vi "CalculoSenoide.vi"(10 "InfoGeraOnda":T1, 11 "InfoOndaIn":cluster{"PontosOnda":dbl[], "IndexTemp":i32}) -> (3 "InfoOndaOut":cluster{"PontosOnda":dbl[], "IndexTemp":i32})   [LabVIEW 2019]
panel:
  # "Max: 60 pontos por segundo"
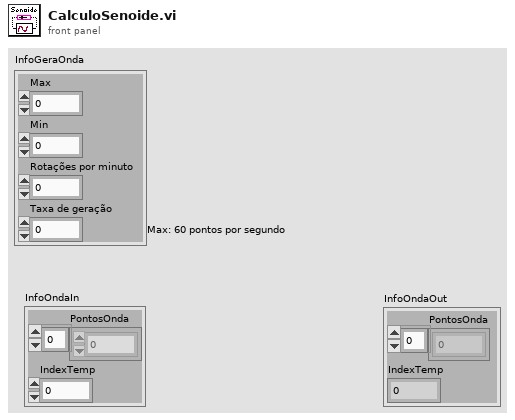
[diagram p1: front panel]
types:
  T1 = cluster{"Max":dbl, "Min":dbl, "Rotações por minuto":dbl, "Taxa de geração":dbl}
  T2 = cluster{"RotaçãoPorSeg":dbl, "Fase":dbl, "AmplitudeOnda":dbl, "Offset":dbl}
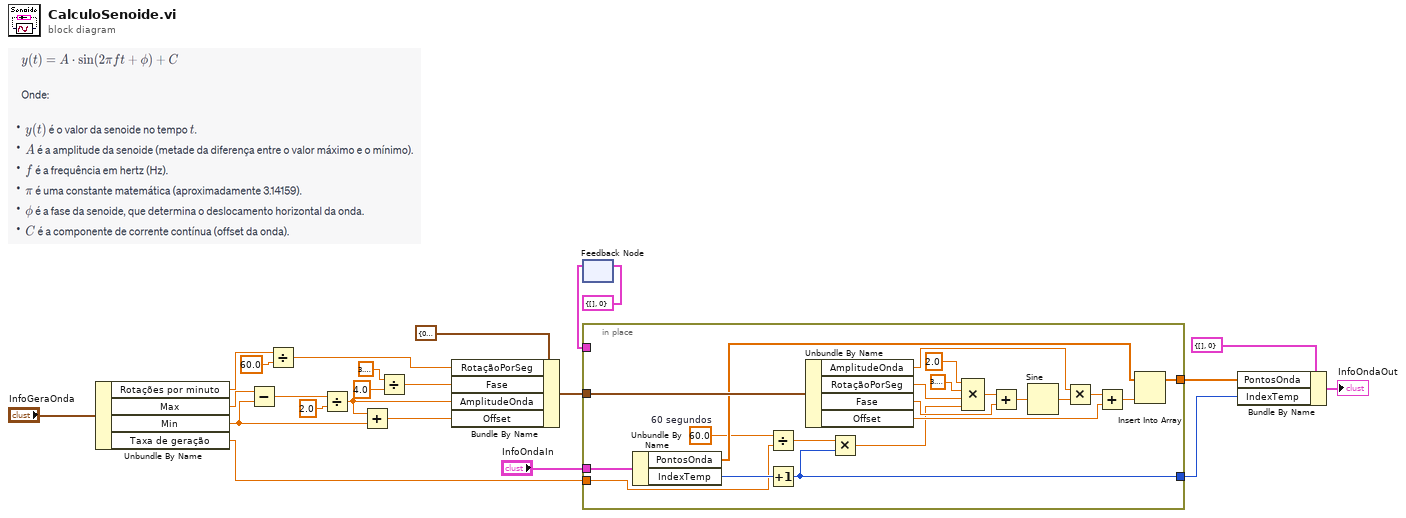
[diagram p0: block diagram]
diagram:
  n1 = Unbundle By Name("InfoGeraOnda") -> ("Rotações por minuto"=w4:dbl, "Max"=w3:dbl, "Min"=w2:dbl, "Taxa de geração"=w1:dbl)
  n2 = Subtract(x=w3, y=w2) -> (x-y=w19:dbl)
  n3 = Divide(x=w4, y=60.0) -> (x/y=w17:dbl)
  n4 = Divide(x=w19, y=2.0) -> (x/y=w15:dbl)
  n5 = Add(x=w15, y=w2) -> (x+y=w14:dbl)
  n6 = Divide(x=3.141592653589793, y=4.0) -> (x/y=w16:dbl)
  n7 = Bundle By Name(cluster=T2 {"RotaçãoPorSeg"=0.0, "Fase"=0.0, "AmplitudeOnda"=0.0, "Offset"=0.0}, "RotaçãoPorSeg"=w17, "Fase"=w16, "AmplitudeOnda"=w15, "Offset"=w14) -> (w13:T2)
  n8 = feedback #1() -> (w12:cluster{"PontosOnda":dbl[], "IndexTemp":i32})  [unwired: 1 in]
  n9 = feedback-in #1(cluster{"PontosOnda":dbl[], "IndexTemp":i32} {"PontosOnda"=[], "IndexTemp"=0}) -> ()
  n10 = in-place {
    in-place-border: w13 -> [w44]
    in-place-border: w12 -> [_]
    in-place-border: [w26] -> w8
    in-place-border: [w27] -> w7
    in-place-border: "InfoOndaIn" -> [w25]
    in-place-border: w1 -> [w24]
    w31 = 60.0  # 60 segundos
    n11 = Unbundle By Name(w25) -> ("PontosOnda"=w43:dbl[], "IndexTemp"=w28:i32)
    n12 = Divide(x=w31, y=w24) -> (x/y=w30:dbl)
    n13 = Increment(x=w28) -> (x+1=w27:i32)
    n14 = Unbundle By Name(w44) -> ("AmplitudeOnda"=w33:dbl, "RotaçãoPorSeg"=w35:dbl, "Fase"=w34:dbl, "Offset"=w32:dbl)
    n15 = Multiply(x=w30, y=w27) -> (x*y=w29:dbl)
    n16 = Compound Arithmetic op=MULTIPLY(2.0, 3.141592653589793, w35, w29) -> (w39:dbl)
    n17 = Add(x=w39, y=w34) -> (x+y=w38:dbl)
    n18 = Sine(x=w38) -> (sin(x)=w40:dbl)
    n19 = Multiply(x=w33, y=w40) -> (x*y=w37:dbl)
    n20 = Add(x=w37, y=w32) -> (x+y=w36:dbl)
    n21 = Insert Into Array(array=w43, new element=w36) -> (w26:dbl[])  [unwired: 1 in]
  }
  n22 = Bundle By Name(cluster=cluster{"PontosOnda":dbl[], "IndexTemp":i32} {"PontosOnda"=[], "IndexTemp"=0} ("InfoOndaIn 2"), "PontosOnda"=w8, "IndexTemp"=w7) -> (→"InfoOndaOut":cluster{"PontosOnda":dbl[], "IndexTemp":i32})
